vi "Get Numeric Type Def Path.vi"(11 "Type":T1) -> (3 "Numeric Type Def Path":path)   [LabVIEW 2016]
uses:
  <vilib>/Utility/Data Type/Type Definitions/Data Type.ctl
  <vilib>/Utility/Data Type/NI_Data Type.lvlib
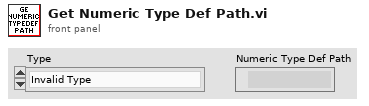
[diagram p1: front panel]
types:
  T1 = typedef "NI_Data Type.lvlib/Data Type.ctl" = enum8{"Invalid Type", "Void", "I8", "I16", "I32", "I64", "U8", "U16", "U32", "U64", "Single Float", "Double Float", "Extended Float", "Single Complex", "Double Complex", "Extended Complex", "Enum U8", "Enum U16", "Enum U32", "Enum U64", "Single Float With Unit", "Double Float With Unit", "Extended Float With Unit", "Single Complex with Unit", "Double Complex with Unit", "Extended Complex with Unit", "Boolean", "String", "Path", "Picture", "Tag", "Array", "Cluster", "Variant", "LV Variant", "Waveform", "Timestamp", "Digital Waveform", "Digital Data", "ExpressData", "Refnum", "External Data", "VI", "Poly VI", "LabVIEW Class Instance", "Fixed Point"}
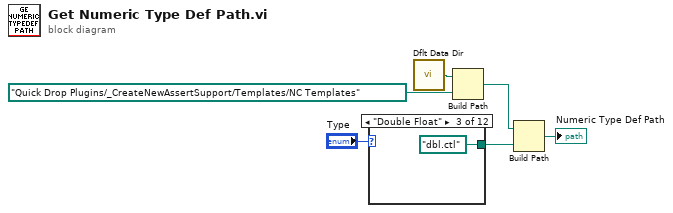
[diagram p0: block diagram]
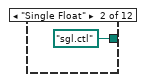
[diagram p3: hidden frame]
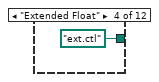
[diagram p4: hidden frame]
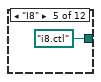
[diagram p5: hidden frame]
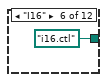
[diagram p6: hidden frame]
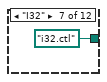
[diagram p7: hidden frame]
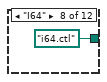
[diagram p8: hidden frame]
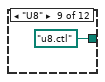
[diagram p9: hidden frame]
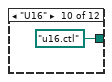
[diagram p10: hidden frame]
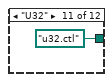
[diagram p11: hidden frame]
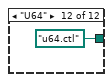
[diagram p12: hidden frame]
diagram:
  n1 = case shown="\"Double Float\"" "Type" {
    tunnel: [_ path "sgl.ctl" ("Path") path "dbl.ctl" ("Path") path "ext.ctl" ("Path") path "i8.ctl" ("Path") path "i16.ctl" ("Path") path "i32.ctl" ("Path") path "i64.ctl" ("Path") path "u8.ctl" ("Path") path "u16.ctl" ("Path") path "u32.ctl" ("Path") path "u64.ctl" ("Path")] -> w3
    frame Default {
    }
    frame "Single Float" {
    }
    frame "Double Float" {
    }
    frame "Extended Float" {
    }
    frame "I8" {
    }
    frame "I16" {
    }
    frame "I32" {
    }
    frame "I64" {
    }
    frame "U8" {
    }
    frame "U16" {
    }
    frame "U32" {
    }
    frame "U64" {
    }
  }
  n2 = call <vilib>:"Dflt Data Dir.vi"() -> ("App:Default Data Directory"=w1:path)
  n3 = Build Path(base path=w1, name or relative path=path "Quick Drop Plugins/_CreateNewAssertSupport/Templates/NC Templates" ("Path")) -> (appended path=w5:path)
  n4 = Build Path(base path=w5, name or relative path=w3) -> (appended path=→"Numeric Type Def Path":path)
